vi "domeADB_logEvent_RotationEnabled.vi"(8 "error in (no error)":errorcluster, 11 "logevent_RotationEnabled_Ctl":T1) -> (0 "error out":errorcluster, 2 "function return":i32, 3 "logevent_RotationEnabled_Ctl out":T1)   [LabVIEW 2016, in "SALLV_domeADB.lvlib"]
doc: "int domeADB_shm_logEvent_RotationEnabledLV(domeADB_logevent_RotationEnabledLV *logevent_RotationEnabled_Ctl );"
uses:
  SALLV_domeADB.lvlib
  DataTypes/logevent_RotationEnabled.ctl
  SALLV_domeADB.so
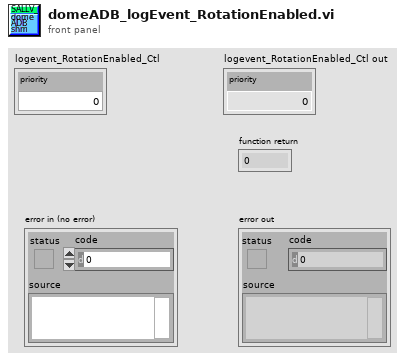
[diagram p1: front panel]
types:
  T1 = typedef "SALLV_domeADB.lvlib/logevent_RotationEnabled.ctl" = cluster{"priority":i32}
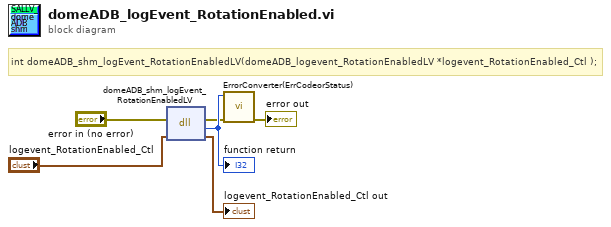
[diagram p0: block diagram]
diagram:
  # "int domeADB_shm_logEvent_RotationEnabledLV(domeADB_logevent_RotationEnabledLV *logevent_RotationEnabled_Ctl );"
  n1 = dll-call lib="home/andres/Desktop/SALLV_domeADB/SALLV_domeADB.*" fn="domeADB_shm_logEvent_RotationEnabledLV"(error in="error in (no error)", "logevent_RotationEnabled_Ctl"="logevent_RotationEnabled_Ctl") -> (error out=w2:errorcluster, w6:i32, "logevent_RotationEnabled_Ctl"=→"logevent_RotationEnabled_Ctl out":T1)  [unwired: 2 in, 1 out]
  "function return" <- w6
  n2 = call "ErrorConverter(ErrCodeorStatus).vi"("error in (no error)"=w2, "error code"=w6) -> ("error out"=→"error out":errorcluster)  [unwired: 9 in]
